vi "Multiply_RGB.vi"(0 "Image Src":T1, 1 "Color Mode":u16(ring) items=["RGB", "HSL", "HSV", "HSI"], 2 "ImageOutput Type":T2 items=["Grayscale (U8)", "Grayscale (I16)", "Grayscale (SGL)", "Complex (CSG)", "RGB (U32)", "HSL (U32)", "RGB (U64)", "Grayscale (U16)"], 5 "R/Hue Image Src":T1, 7 "G/Sat Image Src":T1, 9 "B/Luma/Val Image Src":T1, 11 "error in (no error)":errorcluster, 12 "R/Hue Constant":dbl=1.0 format="%.2f", 13 "G/Sat Constant":dbl=1.0 format="%.2f", 14 "B/Luma/Val Constant":dbl=1.0 format="%.2f") -> (4 "Image Dst Out":T1, 6 "R/Hue Out":T1, 8 "G/Sat Out":T1, 10 "B/Luma/Val Out":T1, 15 "error out":errorcluster)   [LabVIEW 2017]
uses:
  <vilib>/vision/Image Controls.llb/IMAQ Image.ctl
  <vilib>/vision/NI_Vision_Development_Module.lvlib
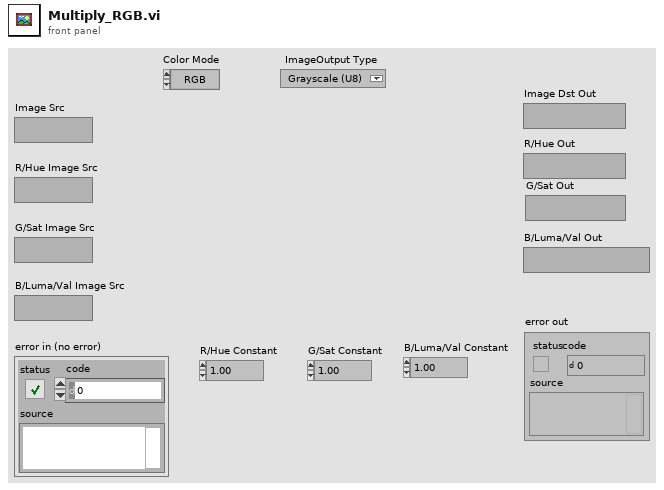
[diagram p1: front panel]
types:
  T1 = typedef "IMAQ Image.ctl" = refnum<image>
  T2 = typedef "Image Type" = u32
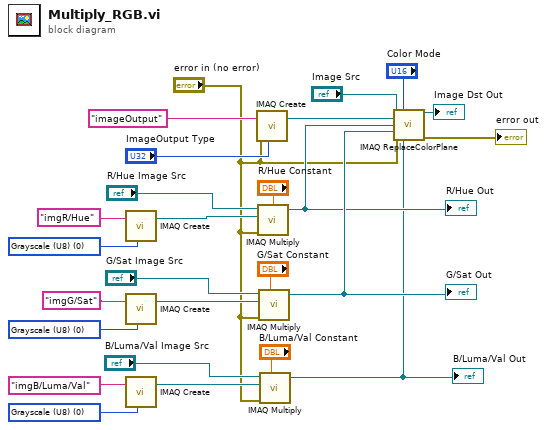
[diagram p0: block diagram]
diagram:
  w8 = T2 0 items=["Grayscale (U8)", "Grayscale (I16)", "Grayscale (SGL)", "Complex (CSG)", "RGB (U32)", "HSL (U32)", "RGB (U64)", "Grayscale (U16)"] ("Image Type")
  w15 = T2 0 items=["Grayscale (U8)", "Grayscale (I16)", "Grayscale (SGL)", "Complex (CSG)", "RGB (U32)", "HSL (U32)", "RGB (U64)", "Grayscale (U16)"] ("Image Type")
  w25 = T2 0 items=["Grayscale (U8)", "Grayscale (I16)", "Grayscale (SGL)", "Complex (CSG)", "RGB (U32)", "HSL (U32)", "RGB (U64)", "Grayscale (U16)"] ("Image Type")
  n1 = call "IMAQ Create"("Image Name"="imgR/Hue", "Image Type"=w15) -> ("New Image"=w14:T1)  [unwired: 3 in, 1 out]
  n2 = call "IMAQ Create"("Image Name"="imgG/Sat", "Image Type"=w25) -> ("New Image"=w24:T1)  [unwired: 3 in, 1 out]
  n3 = call "IMAQ Create"("Image Name"="imgB/Luma/Val", "Image Type"=w8) -> ("New Image"=w7:T1)  [unwired: 3 in, 1 out]
  n4 = call "IMAQ Create"("Image Name"="imageOutput", "Image Type"="ImageOutput Type", "error in (no error)"="error in (no error)") -> ("New Image"=w22:T1)  [unwired: 2 in, 1 out]
  n5 = call "IMAQ Multiply"("Image Src A"="R/Hue Image Src", "Constant"="R/Hue Constant", "Image Dst"=w14, "error in (no error)"="error in (no error)") -> ("Image Dst Out"=w11:T1)  [unwired: 3 in, 1 out]
  "R/Hue Out" <- w11
  n6 = call "IMAQ Multiply"("Image Src A"="G/Sat Image Src", "Constant"="G/Sat Constant", "Image Dst"=w24, "error in (no error)"="error in (no error)") -> ("Image Dst Out"=w21:T1)  [unwired: 3 in, 1 out]
  "G/Sat Out" <- w21
  n7 = call "IMAQ Multiply"("Image Src A"="B/Luma/Val Image Src", "Constant"="B/Luma/Val Constant", "Image Dst"=w7, "error in (no error)"="error in (no error)") -> ("Image Dst Out"=w4:T1)  [unwired: 3 in, 1 out]
  "B/Luma/Val Out" <- w4
  n8 = call "IMAQ ReplaceColorPlane"("Image Src"="Image Src", "Color Mode"="Color Mode", "Image Dst"=w22, "Red or Hue Plane"=w11, "Green or Sat Plane"=w21, "error in (no error)"="error in (no error)", "Blue or Luma or Val or Inten Plane"=w4) -> ("Image Dst Out"=→"Image Dst Out":T1, "error out"=→"error out":errorcluster)  [unwired: 7 in]
